vi "close context.vi"(8 "error in (no error)":errorcluster, 11 "Socket in":refnum<class "Socket2.lvclass">) -> (0 "error out":errorcluster, 3 "Socket out":refnum<class "Socket2.lvclass">)   [LabVIEW 2018, in "Socket2.lvclass"]
uses:
  Socket2.lvclass
  Socket2.lvclass/Socket2.ctl
  <vilib>/addons/zeromq/zmq_context.lvclass
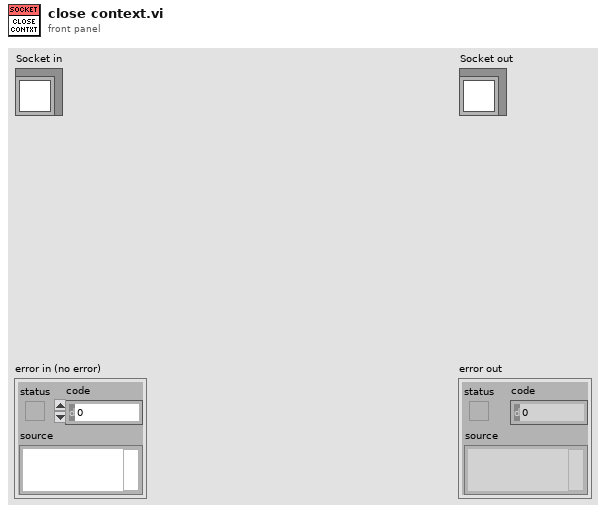
[diagram p1: front panel]
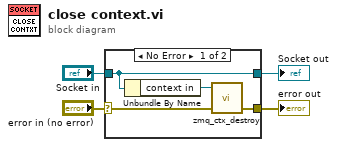
[diagram p0: block diagram]
diagram:
  n1 = case shown="No Error" "error in (no error)" {
    selector: "error in (no error)" -> [w8 w10]
    tunnel: [w7 w10] -> w3
    tunnel: [w6 w9] -> w1
    tunnel: "Socket in" -> [w6 w9]
    frame No Error {
      n2 = Unbundle By Name(w6) -> ("context in"=w5:refnum<class "zmq_context.lvclass">)
      n3 = call <vilib>:"zmq_ctx_destroy.vi"("error in"=w8, "context in"=w5) -> ("error out"=w7:errorcluster)  [unwired: 3 in]
    }
    frame Error {
    }
  }
  "error out" <- w3
  "Socket out" <- w1
